vi "SeqMgr.Initialize Seq, Init Progress Controls.vi"(8 "error in (no error)":errorcluster, 9 "ResultCtrls":T1={"State"=refnum, "Code"=refnum, "Desc"=refnum, "StateColors"=[13816530, 16774304, 16758968, 6618880, 16711680, 16711680, 16711680]}, 10 "ProgressCtrls":T2, 11 "SeqMgr in":refnum<class "SeqMgr.lvclass">) -> (0 "error out":errorcluster, 3 "SeqMgr out":refnum<class "SeqMgr.lvclass">)   [LabVIEW 2024, in "EQMF.lvlib" / "SeqMgr.lvlib" / "SeqMgr.lvclass"]
uses:
  SeqMgr.lvclass
  SeqMgr.Progress Controls.ctl
  SeqMgr.Result Control Ref.ctl
  SeqMgr.Result State Enum.ctl
  SeqMgr.lvclass/SeqMgr.ctl
  SeqMgr.lvlib
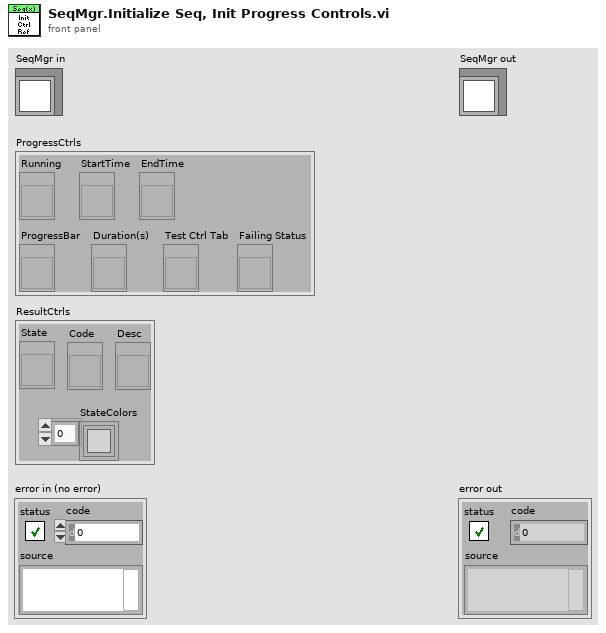
[diagram p1: front panel]
types:
  T1 = typedef "EQMF.lvlib/SeqMgr.lvlib/SeqMgr.Result Control Ref.ctl" = cluster{"State":refnum<vi>, "Code":refnum<vi>, "Desc":refnum<vi>, "StateColors":u32[]}
  T2 = typedef "EQMF.lvlib/SeqMgr.lvlib/SeqMgr.Progress Controls.ctl" = cluster{"Running":refnum<vi>, "StartTime":refnum<vi>, "EndTime":refnum<vi>, "ProgressBar":refnum<vi>, "Duration(s)":refnum<vi>, "Test Ctrl Tab":refnum<vi>, "Failing Status":refnum<vi>}
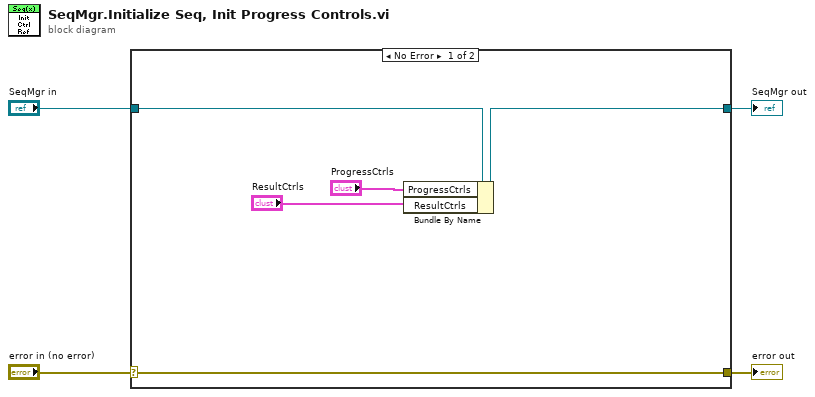
[diagram p0: block diagram]
diagram:
  n1 = case shown="No Error" "error in (no error)" {
    selector: "error in (no error)" -> [w9 w11]
    tunnel: [w9 w11] -> w3
    tunnel: [w7 w10] -> w1
    tunnel: "SeqMgr in" -> [w8 w10]
    frame No Error {
      n2 = Bundle By Name(cluster=w8, "ProgressCtrls"="ProgressCtrls", "ResultCtrls"="ResultCtrls") -> (w7:refnum<class "SeqMgr.lvclass">)
    }
    frame Error {
    }
  }
  "error out" <- w3
  "SeqMgr out" <- w1
